vi "Continue Scan.vi"(8 "error in (no error)":errorcluster, 9 "Feedback State In":T1={"State"=enum."Feedback", "Feedback Parameters"={"Refresh Time (s)"=0.0, "P Gain"=0.0, "Setpoint"=0.0, "Last Update Time"=0.0, "Running average"=0.0, "Points Averaged"=0.0, "Last Average"=0.0, "Filtered signal"=[], "Avging window"=0.0, "Ti"=0.0, "Td"=0.0, "First"=FALSE, "Error Signal Source"=0}, "Scan Parameters"={"Scan Start Time"=0.0, "Step Size (um)"=0.0, "Min Height"=0.0, "Max Height"=0.0, "Dwell Time (s)"=0.0, "Current Step"=0.0}, "Piezo Position"=0.0} {"Feedback Parameters"."Error Signal Source" items=["External Input", "APD Signal"]}, 10 "Feedback Queue":refnum<queue>) -> (0 "error out":errorcluster, 1 "Feedback State Out":T1={"State"=enum."Feedback", "Feedback Parameters"={"Refresh Time (s)"=0.0, "P Gain"=0.0, "Setpoint"=0.0, "Last Update Time"=0.0, "Running average"=0.0, "Points Averaged"=0.0, "Last Average"=0.0, "Filtered signal"=[], "Avging window"=0.0, "Ti"=0.0, "Td"=0.0, "First"=FALSE, "Error Signal Source"=0}, "Scan Parameters"={"Scan Start Time"=0.0, "Step Size (um)"=0.0, "Min Height"=0.0, "Max Height"=0.0, "Dwell Time (s)"=0.0, "Current Step"=0.0}, "Piezo Position"=0.0} {"Feedback Parameters"."Error Signal Source" items=["External Input", "APD Signal"]})   [LabVIEW 2013, in "Feedback.lvlib"]
uses:
  Feedback.lvlib
  support/Message Queue/Message Cluster.ctl
  Feedback State.ctl
  Feedback Parameters.ctl
  Scan Parameters.ctl
  support/Message Queue/Enqueue Message (Single).vi
  support/Message Queue/Message Queue.lvlib
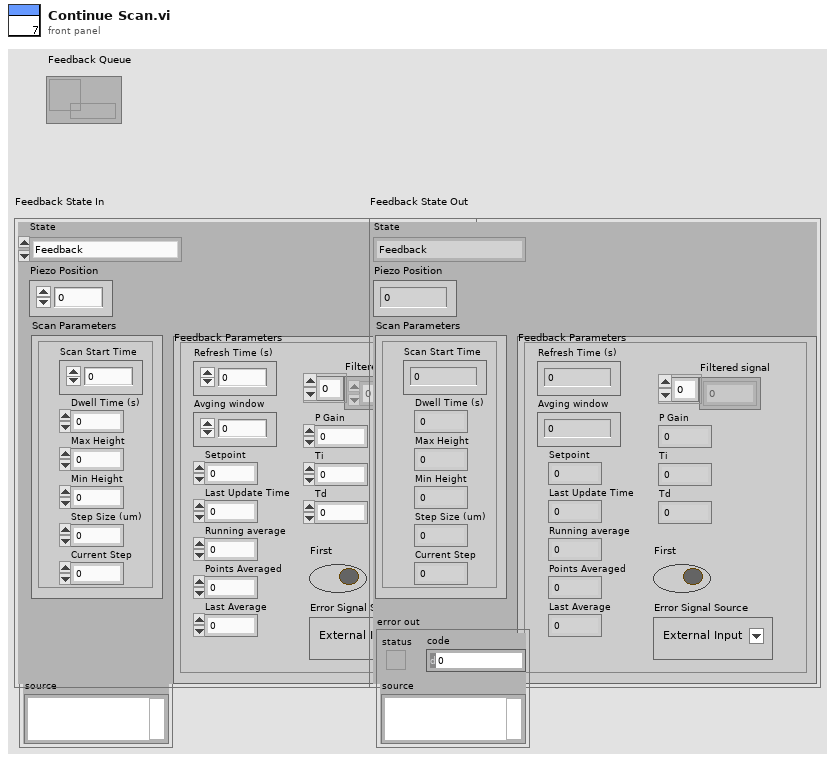
[diagram p1: front panel]
types:
  T1 = typedef "Feedback.lvlib/Feedback State.ctl" = cluster{"State":enum16{"Idle", "Feedback", "Scanning", "Averaging"}, "Feedback Parameters":T2, "Scan Parameters":T3, "Piezo Position":dbl}
  T2 = typedef "Feedback.lvlib/Feedback Parameters.ctl" = cluster{"Refresh Time (s)":dbl, "P Gain":dbl, "Setpoint":dbl, "Last Update Time":dbl, "Running average":dbl, "Points Averaged":dbl, "Last Average":dbl, "Filtered signal":dbl[], "Avging window":dbl, "Ti":dbl, "Td":dbl, "First":bool, "Error Signal Source":u16}
  T3 = typedef "Feedback.lvlib/Scan Parameters.ctl" = cluster{"Scan Start Time":dbl, "Step Size (um)":dbl, "Min Height":dbl, "Max Height":dbl, "Dwell Time (s)":dbl, "Current Step":dbl}
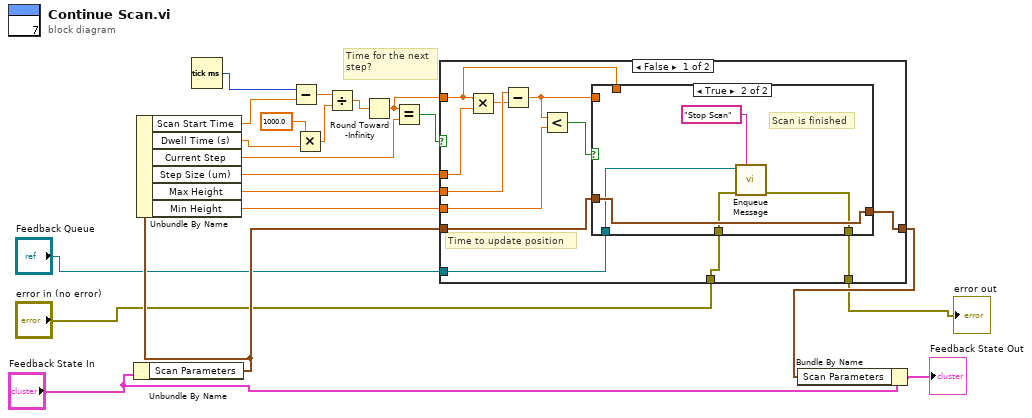
[diagram p0: block diagram]
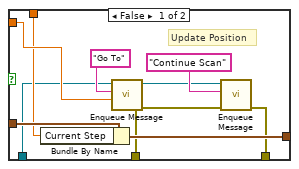
[diagram p2: hidden frame]
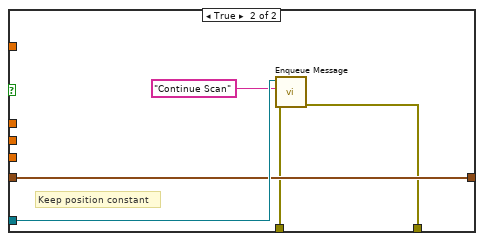
[diagram p3: hidden frame]
diagram:
  # "Time for the next\nstep?"
  n1 = Unbundle By Name("Feedback State In") -> ("Scan Parameters"=w10:T3)
  n2 = Unbundle By Name(w10) -> ("Scan Start Time"=w19:dbl, "Dwell Time (s)"=w8:dbl, "Current Step"=w16:dbl, "Step Size (um)"=w13:dbl, "Max Height"=w12:dbl, "Min Height"=w11:dbl)
  n3 = Tick Count (ms)() -> (millisecond timer value=w20:u32)
  n4 = Subtract(x=w20, y=w19) -> (x-y=w18:dbl)
  n5 = Multiply(x=1000.0, y=w8) -> (x*y=w6:dbl)
  n6 = Divide(x=w18, y=w6) -> (x/y=w17:dbl)
  n7 = Round Toward -Infinity(1:w17) -> (0:w14:dbl)
  n8 = Equal?(x=w14, y=w16) -> (x = y?=w15:bool)
  n9 = case shown="False" w15 {
    tunnel: w14 -> [w22 _]
    tunnel: w13 -> [w32 _]
    tunnel: w12 -> [w31 _]
    tunnel: w11 -> [w28 _]
    tunnel: "Feedback Queue" -> [w21 w52]
    tunnel: [w25 w50] -> w9
    tunnel: w10 -> [w26 w50]
    tunnel: [w24 w49] -> w1
    tunnel: "error in (no error)" -> [w23 w48]
    frame False {
      # "Time to update position"
      n10 = Multiply(x=w22, y=w32) -> (x*y=w30:dbl)
      n11 = Subtract(x=w31, y=w30) -> (x-y=w29:dbl)
      n12 = Less?(x=w29, y=w28) -> (x < y?=w27:bool)
      n13 = case shown="True" w27 {
        tunnel: w29 -> [w40 _]
        tunnel: w26 -> [w39 w46]
        tunnel: [w38 w46] -> w25
        tunnel: [w33 w45] -> w24
        tunnel: w23 -> [w37 w44]
        tunnel: w22 -> [w36 _]
        tunnel: w21 -> [w35 w43]
        frame False {
          # "Update Position"
          n14 = Bundle By Name(cluster=w39, "Current Step"=w36) -> (w38:T3)
          n15 = call-poly "Enqueue Message.vi"("Message Data"=w40, "Message"="Go To", "Message Queue"=w35) -> ("dup Message Queue"=w34:refnum<queue>)  [unwired: 7 in, 1 out]
          n16 = call-poly "Enqueue Message.vi"("error in (no error)"=w37, "Message"="Continue Scan", "Message Queue"=w34) -> ("error out"=w33:errorcluster)  [unwired: 7 in, 1 out]
        }
        frame True {
          # "Scan is finished"
          n17 = call-poly "Enqueue Message.vi"("error in (no error)"=w44, "Message"="Stop Scan", "Message Queue"=w43) -> ("error out"=w45:errorcluster)  [unwired: 7 in, 1 out]
        }
      }
    }
    frame True {
      # "Keep position constant"
      n18 = call-poly "Enqueue Message.vi"("error in (no error)"=w48, "Message"="Continue Scan", "Message Queue"=w52) -> ("error out"=w49:errorcluster)  [unwired: 7 in, 1 out]
    }
  }
  "error out" <- w1
  n19 = Bundle By Name(cluster="Feedback State In", "Scan Parameters"=w9) -> (→"Feedback State Out":T1)
